vi "PRO_Check LevelV1.vi"(8 "Results In in":T3 {"Resistor" format="%.1f"; "Drain" format="%.3f"; "Fill" format="%.3f"}, 9 "Full Cfg":T4, 10 "Measurement":T2, 11 "ChA/!ChB":bool) -> (0 "Results In out":T3 {"Resistor" format="%.1f"; "Drain" format="%.3f"; "Fill" format="%.3f"})   [LabVIEW 2024]
uses:
  Control Definitions/Def FullCfg.ctl
  Control Definitions/Def BenchCfg.ctl
  Control Definitions/Def PumpCtlRefs.ctl
  Control Definitions/Def Bench Status.ctl
  Control Definitions/Def Results2.ctl
  Control Definitions/Def Xresult.ctl
panel:
  out "Indes":i32
  out "Specs":dbl[](array[numeric])
  out "Status":T1
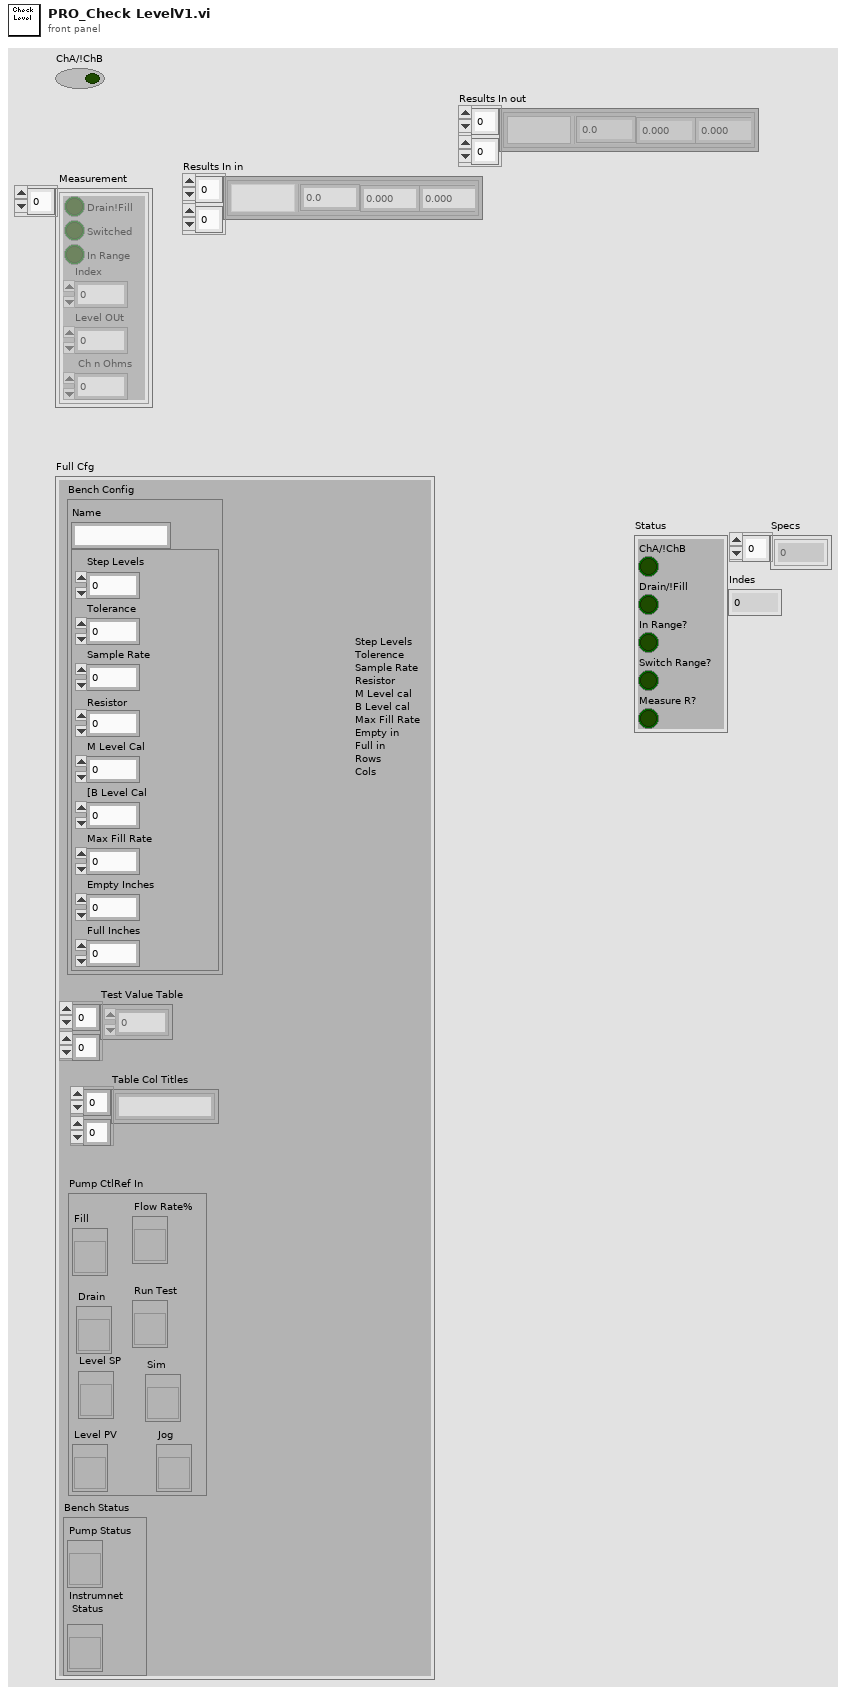
[diagram p1: front panel]
types:
  T1 = cluster{"ChA/!ChB":bool, "Drain/!Fill":bool, "In Range?":bool, "Switch Range?":bool, "Measure R?":bool}
  T2 = typedef "Def Xresult.ctl" = cluster{"Switched":bool, "In Range":bool, "Index":i16, "Level OUt":dbl, " Ch n Ohms":dbl, "Drain!Fill":bool}[]
  T3 = typedef "Def Results2.ctl" = cluster{"Fill":dbl, "Drain":dbl, "Status":i16, "Resistor":dbl}[][]
  T4 = typedef "Def FullCfg.ctl" = cluster{"Bench Config":T5, "Test Value Table ":dbl[][], "Table Col Titles":string[][], "Pump CtlRef In":T6, "Bench Status":T7}
  T5 = typedef "Def BenchCfg.ctl" = cluster{"Name":string, cluster{"Step Levels":dbl, "Tolerance":dbl, "Sample Rate":dbl, "Resistor":dbl, "M Level Cal":dbl, "[B Level Cal":dbl, "Max Fill Rate":dbl, "Empty Inches":dbl, "Full Inches":dbl}}
  T6 = typedef "Def PumpCtlRefs.ctl" = cluster{"Fill ":refnum<vi>, "Drain":refnum<vi>, "Level PV":refnum<vi>, "Flow Rate%":refnum<vi>, "Run Test":refnum<vi>, "Sim":refnum<vi>, "Jog":refnum<vi>, "Level SP":refnum<vi>}
  T7 = typedef "Def Bench Status.ctl" = cluster{"Pump Status":refnum<vi>, "Instrumnet\n Status":refnum<vi>}
  T8 = cluster{"Switched":bool, "In Range":bool, "Index":i16, "Level OUt":dbl, " Ch n Ohms":dbl, "Drain!Fill":bool}
  T9 = cluster{"Fill":dbl, "Drain":dbl, "Status":i16, "Resistor":dbl}
  T10 = typedef "Ded Spec RNG.ctl" = cluster{"Specs":dbl[], "Indes":i32, "LUT Status":T11}
  T11 = typedef "Ded LUT_Status.ctl" = cluster{"ChA/!ChB":bool, "Drain/!Fill":bool, "In Range?":bool, "Switch Range?":bool, "Measure R?":bool, "Vaild R?":bool}
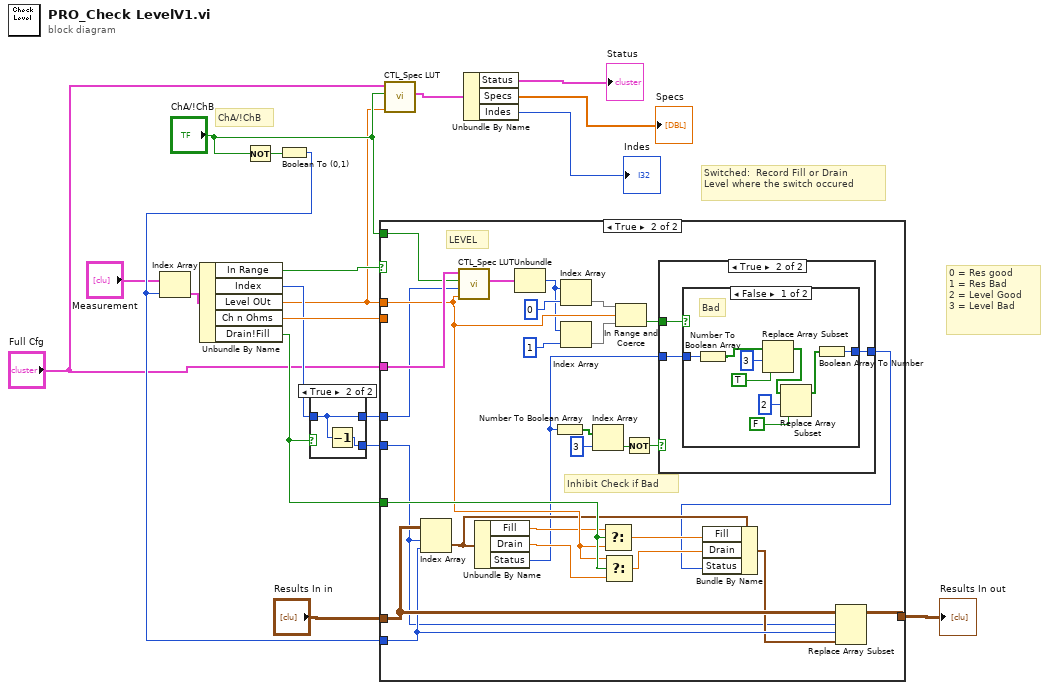
[diagram p0: block diagram]
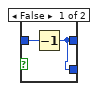
[diagram p2: hidden frame]
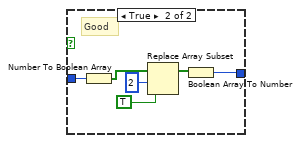
[diagram p5: hidden frame]
diagram:
  # "0 = Res good\n1 = Res Bad\n2 = Level Good\n3 = Level Bad"
  # "Switched:  Record Fill or Drain\nLevel where the switch occured"
  # "ChA/!ChB"
  n1 = Not(x="ChA/!ChB") -> (.not. x?=w19:bool)
  n2 = Boolean To (0,1)(Boolean=w19) -> (0, 1=w18:i16)
  n3 = Index Array(array="Measurement", index=w18) -> (element=w13:T8)
  n4 = Unbundle By Name(w13) -> ("In Range"=w17:bool, "Index"=w10:i16, "Level OUt"=w1:dbl, "Ch n Ohms"=w16:dbl, "Drain!Fill"=w11:bool)
  n5 = case shown="True" w11 {
    tunnel: w10 -> [w21 w23]
    tunnel: [w20 w23] -> w9
    tunnel: [w20 w22] -> w8
    frame False {
      n6 = Decrement(x=w21) -> (x-1=w20:i16)
    }
    frame True {
      n7 = Decrement(x=w23) -> (x-1=w22:i16)
    }
  }
  n8 = case shown="True" w17 {
    tunnel: "Full Cfg" -> [_ w48]
    tunnel: [w24 w52] -> w14
    tunnel: "Results In in" -> [w24 w51]
    tunnel: w1 -> [_ w43]
    tunnel: w16 -> [_ _]
    tunnel: w11 -> [_ w50]
    tunnel: w18 -> [_ w49]
    tunnel: "ChA/!ChB" -> [_ w35]
    tunnel: w9 -> [_ w27]
    tunnel: w8 -> [_ w26]
    frame False {
    }
    frame True {
      # "Inhibit Check if Bad"
      # "LEVEL"
      n9 = Index Array(array=w51, index (row)=w26, index (col)=w49) -> (element=w39:T9)
      n10 = call "CTL_Spec LUT.vi"("Level IN inches"=w43, "Index"=w27, "ChA/!ChB"=w35, "Full Cfg"=w48) -> ("Spec RNG"=w47:T10)  [unwired: 4 in, 3 out]
      n11 = Unbundle By Name(w39) -> ("Fill"=w41:dbl, "Drain"=w40:dbl, "Status"=w29:i16)
      n12 = Unbundle(w47) -> ("Indes"=w25:i32)  [unwired: 2 out]
      n13 = Number To Boolean Array(number=w29) -> (Boolean array=w32:bool[])
      n14 = Index Array(array=w25, index=0) -> (element=w44)
      n15 = Index Array(array=w25, index=1) -> (element=w45)
      n16 = Index Array(array=w32, index=3) -> (element=w30:bool)
      n17 = Select(t=w41, s=w50, f=w43) -> (s? t:f=w37:dbl)
      n18 = Select(t=w43, s=w50, f=w40) -> (s? t:f=w36:dbl)
      n19 = In Range and Coerce(upper limit=w44, x=w43, lower limit=w45) -> (In Range?=w34:bool)  [unwired: 1 out]
      n20 = Not(x=w30) -> (.not. x?=w28:bool)
      n21 = case shown="True" w28 {
        tunnel: w34 -> [_ w56]
        tunnel: [w53 w55] -> w33
        tunnel: w29 -> [w53 w54]
        frame False {
        }
        frame True {
          n22 = case shown="False" w56 {
            tunnel: w54 -> [w63 w69]
            tunnel: [w61 w66] -> w55
            frame False {
              # "Bad"
              n23 = Number To Boolean Array(number=w63) -> (Boolean array=w62:bool[])
              n24 = Replace Array Subset(array=w62, new element=TRUE ("new element/subarray"), index=3) -> (w58:bool[])
              n25 = Replace Array Subset(array=w58, new element=FALSE ("new element/subarray"), index=2) -> (w57:bool[])
              n26 = Boolean Array To Number(Boolean array=w57) -> (number=w61:u32)
            }
            frame True {
              # "Good"
              n27 = Number To Boolean Array(number=w69) -> (Boolean array=w68:bool[])
              n28 = Replace Array Subset(array=w68, new element=TRUE ("new element/subarray"), index=2) -> (w67:bool[])
              n29 = Boolean Array To Number(Boolean array=w67) -> (number=w66:u32)
            }
          }
        }
      }
      n30 = Bundle By Name(cluster=w39, "Fill"=w37, "Drain"=w36, "Status"=w33) -> (w38:T9)
      n31 = Replace Array Subset(array=w51, new element=w38, index (row)=w26, index (col)=w49) -> (w52:T3)
    }
  }
  "Results In out" <- w14
  n32 = call "CTL_Spec LUT.vi"("Level IN inches"=w1, "ChA/!ChB"="ChA/!ChB", "Full Cfg"="Full Cfg") -> ("Spec RNG"=w5:T10)  [unwired: 5 in, 3 out]
  n33 = Unbundle By Name(w5) -> ("Status"=→"Status":T1, "Specs"=→"Specs":dbl[], "Indes"=→"Indes":i32)
